vi "VFD Ramp Calculation.vi"(11 "element":dbl) -> (2 "intercept 7":dbl, 3 "slope 7":dbl)   [LabVIEW 2018]
uses:
  <vilib>/Analysis/1siggen.llb/Ramp Pattern by Samples.vi
  <vilib>/Analysis/NI_AALBase.lvlib
  <vilib>/Analysis/NI_AALPro.lvlib
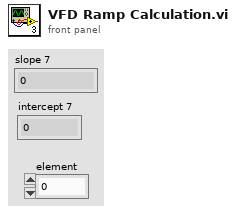
[diagram p1: front panel]
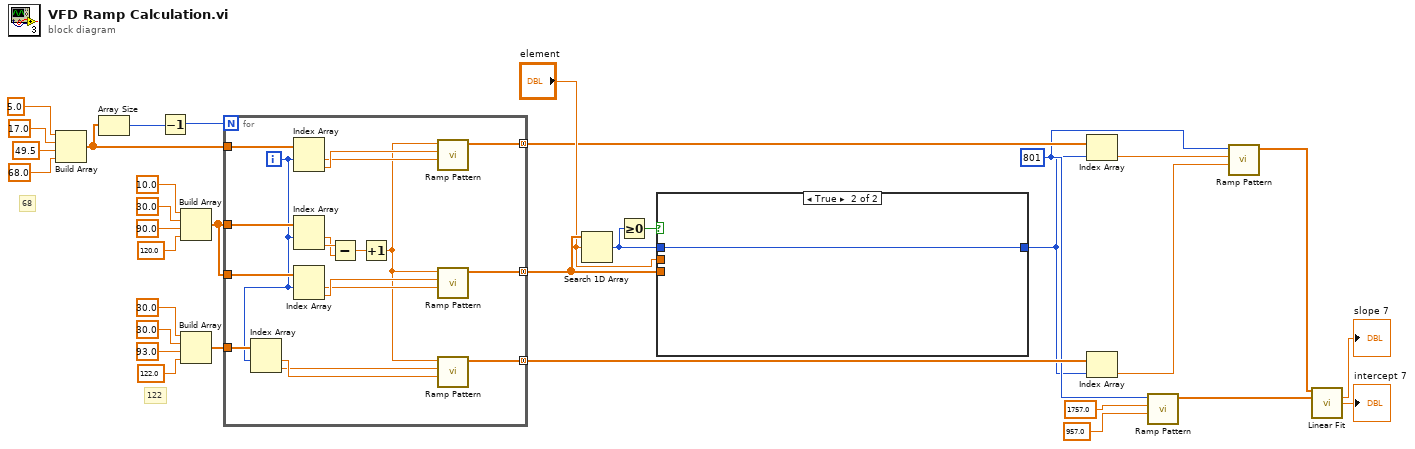
[diagram p0: block diagram]
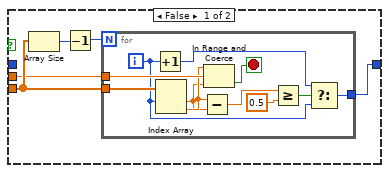
[diagram p2: hidden frame]
diagram:
  w10 = 801 ("samples")
  # "68"
  # "122"
  n1 = Build Array(5.0 ("end"), 17.0 ("end"), 49.5 ("end"), 68.0 ("end")) -> (w21:dbl[])
  n2 = Array Size(array=w21) -> (size(s)=w23:i32)
  n3 = Decrement(x=w23) -> (x-1=w22:i32)
  n4 = Build Array(10.0 ("element"), 30.0 ("element"), 90.0 ("element"), 120.0 ("element")) -> (w19:dbl[])
  n5 = Build Array(30.0 ("start"), 30.0 ("start"), 93.0 ("start"), 122.0 ("start")) -> (w20:dbl[])
  n6 = for {
    N: w22 -> [_]
    tunnel: w21 -> [w47]
    tunnel: w20 -> [w42]
    tunnel: w19 -> [w51]
    tunnel: [w48] -> w14 mode=concatenating
    tunnel: [w41] -> w13 mode=concatenating
    tunnel: w19 -> [w38]
    tunnel: [w36] -> w17 mode=concatenating
    i -> [w34]
    n7 = Index Array(array=w42, index #1=w34) -> (element #1=w44:dbl, element #2=w43:dbl)  [unwired: 1 in]
    n8 = Index Array(array=w47, index #1=w34) -> (element #1=w45:dbl, element #2=w46:dbl)  [unwired: 1 in]
    n9 = Index Array(array=w51, index #1=w34) -> (element #1=w49:dbl, element #2=w50:dbl)  [unwired: 1 in]
    n10 = Index Array(array=w38, index #1=w34) -> (element #1=w39:dbl, element #2=w40:dbl)  [unwired: 1 in]
    n11 = Subtract(x=w50, y=w49) -> (x-y=w37:dbl)
    n12 = Increment(x=w37) -> (x+1=w35:dbl)
    n13 = call-poly <vilib>:"Ramp Pattern.vi"("start"=w45, "end"=w46, "samples"=w35) -> ("Ramp Pattern"=w48:dbl[])  [unwired: 7 in, 1 out]
    n14 = call-poly <vilib>:"Ramp Pattern.vi"("start"=w39, "end"=w40, "samples"=w35) -> ("Ramp Pattern"=w36:dbl[])  [unwired: 7 in, 1 out]
    n15 = call-poly <vilib>:"Ramp Pattern.vi"("start"=w44, "end"=w43, "samples"=w35) -> ("Ramp Pattern"=w41:dbl[])  [unwired: 7 in, 1 out]
  }
  n16 = Search 1D Array(1D array=w17, element="element") -> (index of element=w15:i32)  [unwired: 1 in]
  n17 = Greater Or Equal To 0?(x=w15) -> (x >= 0?=w18:bool)
  n18 = case shown="True" w18 {
    tunnel: w17 -> [w54 _]
    tunnel: "element" -> [w53 _]
    tunnel: [w52 w68] -> w5
    tunnel: w15 -> [_ w68]
    frame False {
      n19 = Array Size(array=w54) -> (size(s)=w56:i32)
      n20 = Decrement(x=w56) -> (x-1=w55:i32)
      n21 = for {
        N: w55 -> [_]
        tunnel: w54 -> [w67]
        tunnel: w53 -> [w66]
        tunnel: [w58] -> w52
        i -> [w60]
        stop <- w57 stop-if-true
        n22 = Increment(x=w60) -> (x+1=w59:i32)
        n23 = Index Array(array=w67, index #1=w60) -> (element #1=w61:dbl, element #2=w62:dbl)  [unwired: 1 in]
        n24 = Subtract(x=w62, y=w61) -> (x-y=w65:dbl)
        n25 = In Range and Coerce(upper limit=w62, x=w66, lower limit=w61) -> (In Range?=w57:bool)  [unwired: 1 out]
        n26 = Greater Or Equal?(x=w65, y=0.5) -> (x >= y?=w63:bool)
        n27 = Select(t=w59, s=w63, f=w60) -> (s? t:f=w58:i32)
      }
    }
    frame True {
    }
  }
  n28 = Index Array(array=w14, index=w5) -> (element=w2:dbl)
  n29 = Index Array(array=w13, index=w5) -> (element=w1:dbl)
  n30 = call-poly <vilib>:"Ramp Pattern.vi"("start"=957.0, "end"=1757.0, "samples"=w10) -> ("Ramp Pattern"=w8:dbl[])  [unwired: 7 in, 1 out]
  n31 = call-poly <vilib>:"Ramp Pattern.vi"("start"=w1, "end"=w2, "samples"=w10) -> ("Ramp Pattern"=w9:dbl[])  [unwired: 7 in, 1 out]
  n32 = call <vilib>:"Linear Fit.vi"("Y"=w9, "X"=w8) -> ("slope"=→"slope 7":dbl, "intercept"=→"intercept 7":dbl)  [unwired: 9 in, 3 out]
